vi "Import Modbus CSV Map.vi"(11 "CSV Test File Path":path) -> (3 "Modbus address map":T4(array[cluster]))   [LabVIEW 2013, in "Modbus Slave tests.lvlib"]
uses:
  <vilib>/NI/Tag Bus Module Framework/channel/channel classification.ctl
  <vilib>/NI/Tag Bus/tag/Data Type.ctl
  module channel/data bank type.ctl
  <vilib>/Utility/file.llb/Read From Spreadsheet File (string).vi
  Modbus Slave tests.lvlib
  <vilib>/NI/Tag Bus Module Framework/channel/TBM channel.lvclass
  <vilib>/NI/Tag Bus/tag/tag descriptor.lvclass
  module channel/Modbus Module Channel.lvclass
panel:
  out "all rows":string[][](array[string])
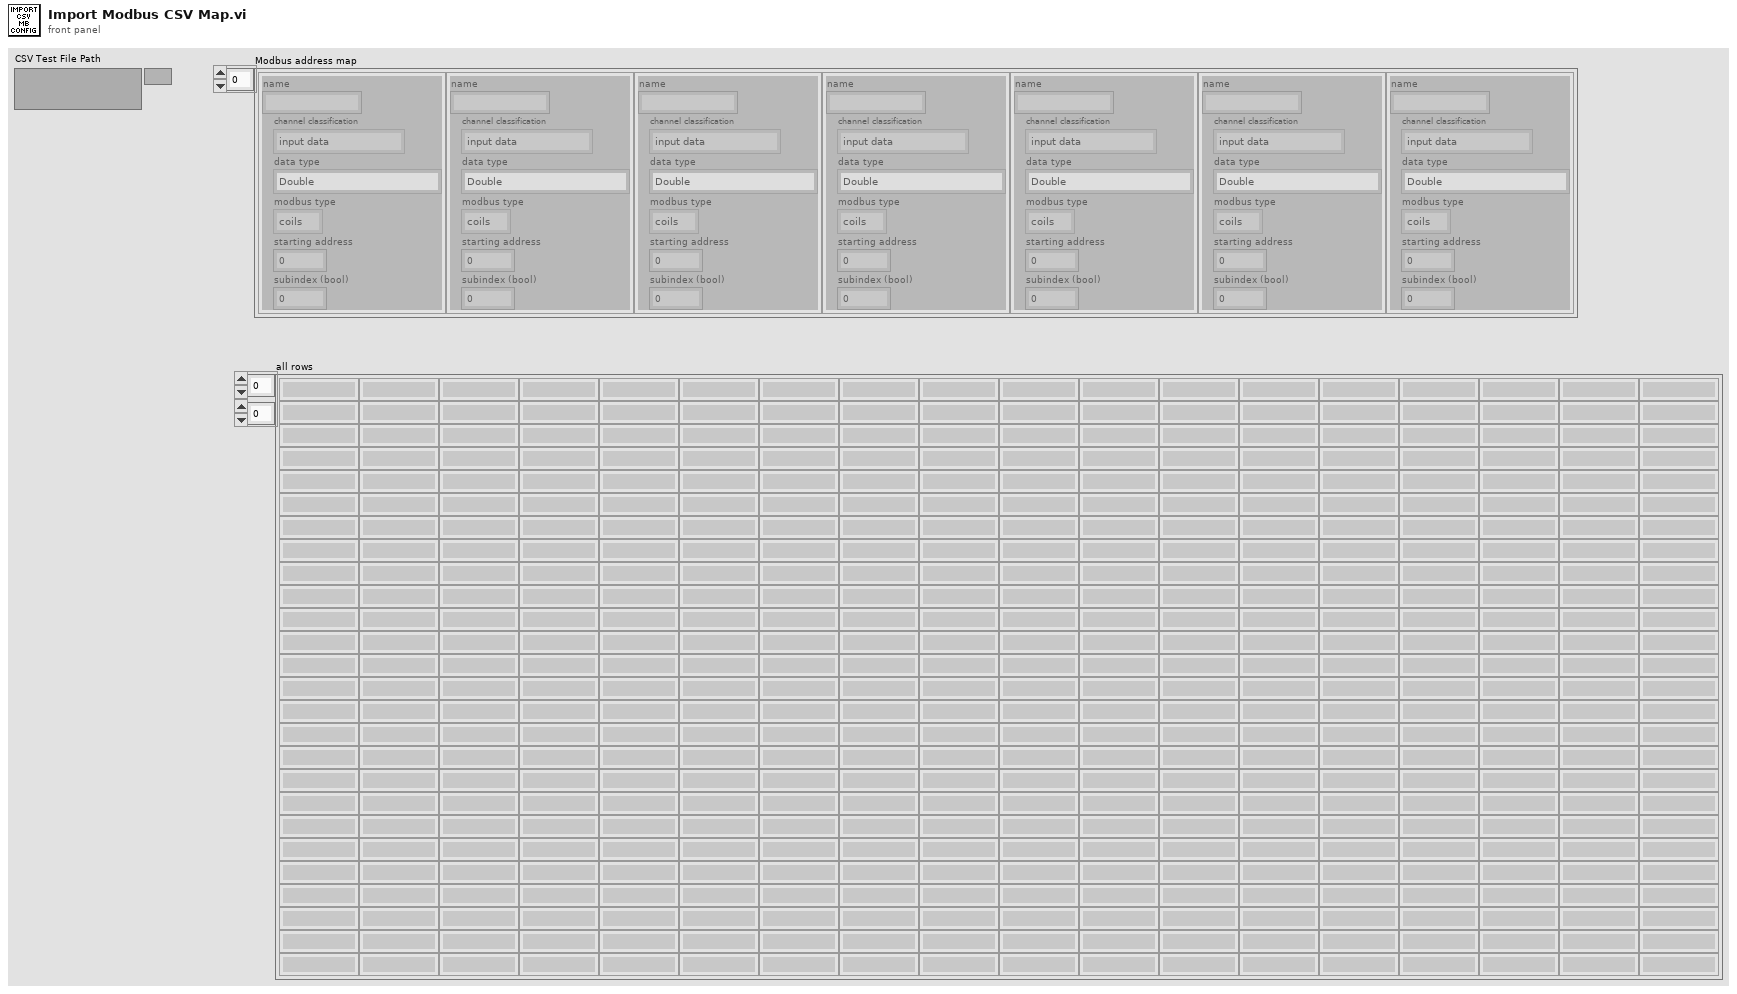
[diagram p1: front panel]
types:
  T1 = typedef "TBM channel.lvclass/channel classification.ctl" = enum16{"input data", "output data", "processing parameter", "processing result"}
  T2 = typedef "tag bus.lvlib/tag descriptor.lvclass/Data Type.ctl" = enum16{"Double", "Single", "I64", "I32", "I16", "I8", "U64", "U32", "U16", "U8", "Boolean", "String", "Array of Double", "Array of Single", "Array of I64", "Array of I32", "Array of I16", "Array of I8", "Array of U64", "Array of U32", "Array of U16", "Array of U8", "Array of Boolean", "Array of String"}
  T3 = typedef "Modbus Module Channel.lvclass/data bank type.ctl" = enum16{"coils", "discrete inputs", "input registers", "holding registers"}
  T4 = cluster{"name":string, "channel classification":T1, "data type":T2, "modbus type":T3, "starting address":u16, "subindex (bool)":i32}[]
  T5 = cluster{"name":string, "channel classification":T1, "data type":T2, "modbus type":T3, "starting address":u16, "subindex (bool)":i32}
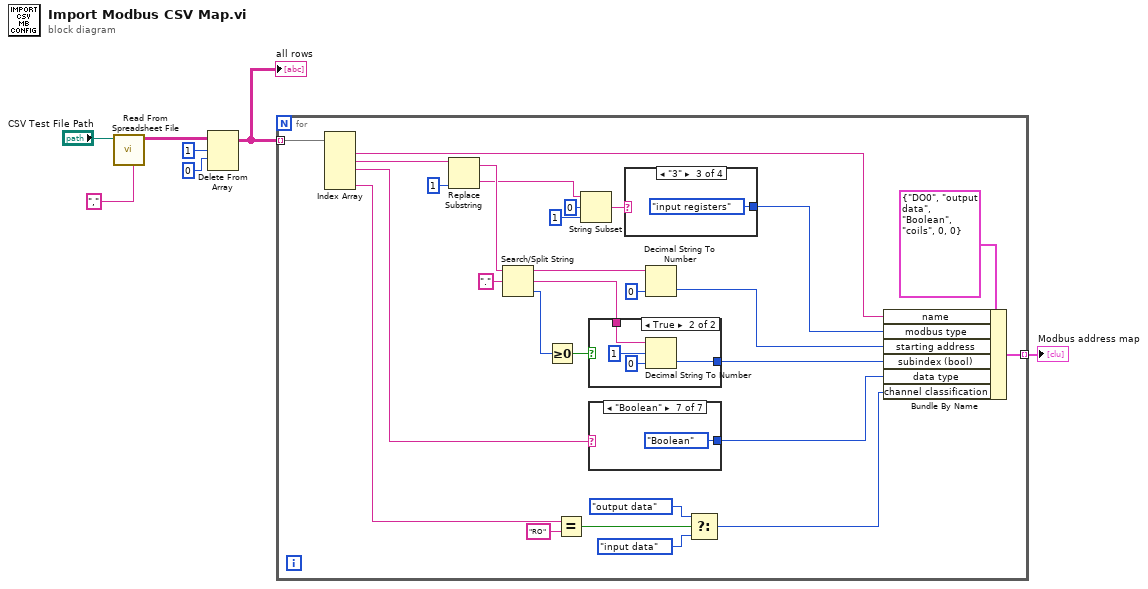
[diagram p0: block diagram]
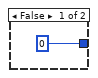
[diagram p2: hidden frame]
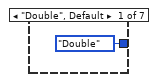
[diagram p3: hidden frame]
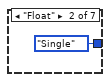
[diagram p4: hidden frame]
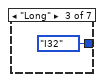
[diagram p5: hidden frame]
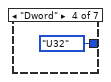
[diagram p6: hidden frame]
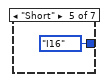
[diagram p7: hidden frame]
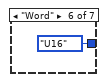
[diagram p8: hidden frame]
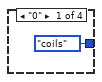
[diagram p9: hidden frame]
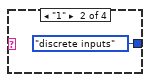
[diagram p10: hidden frame]
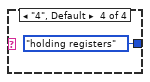
[diagram p11: hidden frame]
diagram:
  n1 = call-poly <vilib>:"Read From Spreadsheet File.vi"("delimiter (\\t)"="," ("delimiter (\\t)"), "file path (dialog if empty)"="CSV Test File Path") -> ("all rows"=w4:string[][])  [unwired: 5 in, 4 out]
  n2 = Delete From Array(array=w4, length=1, index (row)=0) -> (array with subset deleted=w3:string[][])  [unwired: 1 in, 1 out]
  "all rows" <- w3
  n3 = for {
    tunnel: w3 -> [w35] mode=indexing
    tunnel: [w11] -> w5 mode=indexing
    n4 = Index Array(array=w35) -> (element #1=w33:string, element #2=w20:string, element #3=w29:string, element #5=w27:string)  [unwired: 5 in, 1 out]
    n5 = Replace Substring(2:1 ("length (len. of substring)"), 5:w20) -> (0:w17:string, 1:w18:string)  [unwired: 2 in]
    n6 = Search/Split String(string=w18, search string/char (-)=".") -> (substring before match=w15:string, match + rest of string=w13:string, offset of match=w8:i32)  [unwired: 1 in]
    n7 = Greater Or Equal To 0?(x=w8) -> (x >= 0?=w10:bool)
    n8 = Equal?(x=w27, y="RO") -> (x = y?=w23:bool)
    n9 = String Subset(string=w17, offset (0)=0, length (rest)=1 ("length (rest)")) -> (substring=w31:string)
    n10 = case shown="True" w10 {
      tunnel: w13 -> [_ w39]
      tunnel: [0 w38] -> w12
      frame False {
      }
      frame True {
        n11 = Decimal String To Number(string=w39, offset=1, default (0L)=0 ("subindex (bool)")) -> (number=w38:i32)  [unwired: 1 out]
      }
    }
    n12 = case shown="\"Boolean\"" w29 {
      tunnel: [Data_Type."Double" ("data type") Data_Type."Single" ("data type") Data_Type."I32" ("data type") Data_Type."U32" ("data type") Data_Type."I16" ("data type") Data_Type."U16" ("data type") Data_Type."Boolean" ("data type")] -> w28
      frame "Double", Default {
      }
      frame "Float" {
      }
      frame "Long" {
      }
      frame "Dword" {
      }
      frame "Short" {
      }
      frame "Word" {
      }
      frame "Boolean" {
      }
    }
    n13 = case shown="\"3\"" w31 {
      tunnel: [data_bank_type."coils" ("modbus type") data_bank_type."discrete inputs" ("modbus type") data_bank_type."input registers" ("modbus type") data_bank_type."holding registers" ("modbus type")] -> w30
      frame "0" {
      }
      frame "1" {
      }
      frame "3" {
      }
      frame "4", Default {
      }
    }
    n14 = Decimal String To Number(string=w15, default (0L)=u16 0 ("starting address")) -> (number=w9:u16)  [unwired: 1 in, 1 out]
    n15 = Select(t=channel_classification."output data" ("channel classification"), s=w23, f=channel_classification."input data" ("channel classification")) -> (s? t:f=w22:T1)
    n16 = Bundle By Name(cluster=T5 {"name"="DO0", "channel classification"=enum."output data", "data type"=enum."Boolean", "modbus type"=enum."coils", "starting address"=0, "subindex (bool)"=0}, "name"=w33, "modbus type"=w30, "starting address"=w9, "subindex (bool)"=w12, "data type"=w28, "channel classification"=w22) -> (w11:T5)
  }
  "Modbus address map" <- w5
